vi "receivedMessage.vi"(8 "error in (no error)":errorcluster, 10 "message":string, 11 "TCPComEvents in":refnum<class "TCPComEvents.lvclass">) -> (0 "error out":errorcluster, 3 "TCPComEvents out":refnum<class "TCPComEvents.lvclass">)   [LabVIEW 2016, in "TCPComEvents.lvclass"]
uses:
  TCPComEvents.lvclass
  TCPComEvents.lvclass/TCPComEvents.ctl
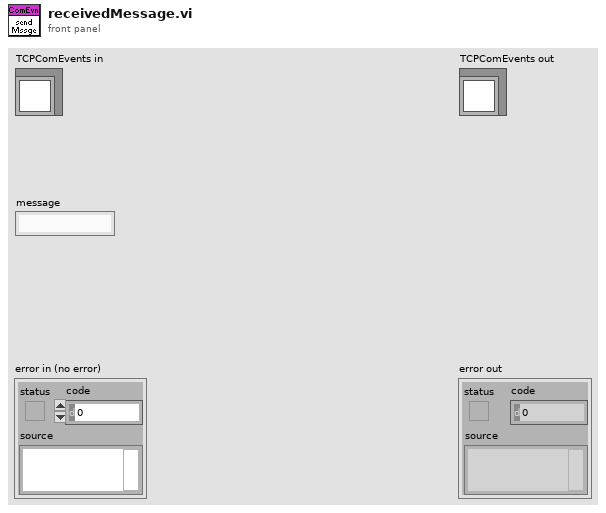
[diagram p1: front panel]
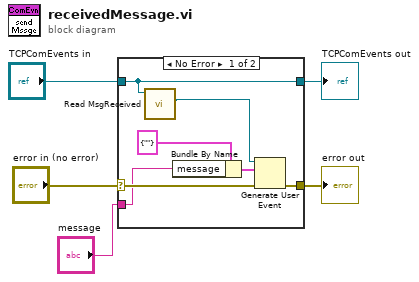
[diagram p0: block diagram]
diagram:
  n1 = case shown="No Error" "error in (no error)" {
    selector: "error in (no error)" -> [w12 w14]
    tunnel: [w11 w14] -> w4
    tunnel: [w7 w13] -> w2
    tunnel: "TCPComEvents in" -> [w7 w13]
    tunnel: "message" -> [w8 _]
    frame No Error {
      n2 = call "Read MsgReceived.vi"("TCPComEvents in"=w7) -> ("MsgReceived"=w6:refnum<user-event>)  [unwired: 8 in, 2 out]
      n3 = Bundle By Name(cluster=cluster{"message":string} {"message"=""} ("event data"), "message"=w8) -> (w9:cluster{"message":string})
      n4 = Generate User Event(user event=w6, event data cluster=w9, error in=w12) -> (error out=w11:errorcluster)  [unwired: 1 in, 1 out]
    }
    frame Error {
    }
  }
  "error out" <- w4
  "TCPComEvents out" <- w2
